vi "Save Displayed Image.vi"(8 "error in (no error)":errorcluster, 9 "Saved Image File Format":T2, 10 "File Path in":path, 11 "Display Image Control Refnum":T1) -> (0 "Error Out":errorcluster, 2 "File Path out":path)   [LabVIEW 2021]
uses:
  Pictures/Save File Format.ctl
  Image Control Refnum.ctl
  Selected Area in Object.ctl
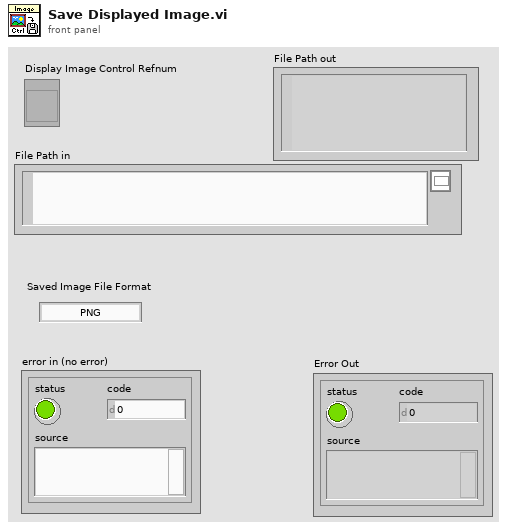
[diagram p1: front panel]
types:
  T1 = typedef "Image Control Refnum.ctl" = refnum<vi>
  T2 = typedef "Save File Format.ctl" = enum16{"PNG", "JPEG", "BMP"}
  T3 = typedef "Selected Area in Object.ctl" = cluster{"Selected Area Position Left":i32, "Selected Area Position Top":i32, "Selected Area Size Height":u32, "Selected Area Size Width":u32, "Object Position Left":i32, "Object Position Top":i32}
  T4 = typedef "imagedata.ctl" = cluster{"image type":i32, "image depth":i32, "image":u8[], "mask":u8[], "colors":u32[], "Rectangle":cluster{"left":i16, "top":i16, "right":i16, "bottom":i16}}
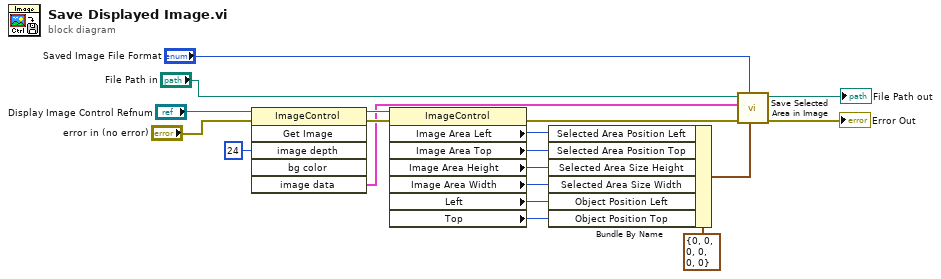
[diagram p0: block diagram]
diagram:
  n1 = invoke class="ImageControl" method="Get Image"(reference="Display Image Control Refnum", error in="error in (no error)", "image depth"=24 ("Image Depth")) -> (reference out=w16:T1, error out=w14:errorcluster, "image data"=w2:T4)  [unwired: 3 in, 3 out]
  n2 = property class="ImageControl"(reference=w16, error in=w14) -> (error out=w13:errorcluster, "Image Area Left"=w10:i32, "Image Area Top"=w9:i32, "Image Area Height"=w8:u32, "Image Area Width"=w7:u32, "Left"=w6:i32, "Top"=w5:i32)  [unwired: 1 out]
  n3 = Bundle By Name(cluster=T3 {"Selected Area Position Left"=0, "Selected Area Position Top"=0, "Selected Area Size Height"=0, "Selected Area Size Width"=0, "Object Position Left"=0, "Object Position Top"=0} ("output cluster"), "Selected Area Position Left"=w10, "Selected Area Position Top"=w9, "Selected Area Size Height"=w8, "Selected Area Size Width"=w7, "Object Position Left"=w6, "Object Position Top"=w5) -> (w3:T3)
  n4 = call "Save Selected Area in Image.vi"("Selected Area in Object"=w3, "Saved Image File Format"="Saved Image File Format", "error in (no error)"=w13, "Image Data"=w2, "File Path in"="File Path in") -> ("error out"=→"Error Out":errorcluster, "File Path out"=→"File Path out":path)  [unwired: 5 in]
